vi "Teleop.vi"(10 "Match Info":T1={"Autonomous Elapsed Seconds"=0.0, "TeleOp Elapsed Seconds"=0.0, "Disabled Elapsed Seconds"=0.0, "Visited Autonomous"=FALSE, "Visited TeleOp"=FALSE, "Visited Disabled"=FALSE, "Autonomous Settings"={"Autonomous Style"=enum."Independent", "VI Refnum"=refnum}}, 11 "Call Context":T2) -> ()   [LabVIEW 2017]
doc: "This VI is called for each enabled TeleOp packet received from the DS. It is typically used to read from joysticks and other inputs and update I/O or setpoints for timed control loops. It should complete and return within 20 milliseconds or risk missing DS packets."
uses:
  <vilib>/Rock Robotics/WPI/DriverStation/WPI_DriverStationDerivedRobotMode.ctl
  <vilib>/Rock Robotics/WPI/DriverStation/WPI_DriverStationMatch Info.ctl
  <vilib>/Rock Robotics/WPI/Utilities/WPI_GetSetVariantRefNum.vi
  <vilib>/Rock Robotics/Network Tables/NT Write Boolean Array.vi
  <vilib>/Rock Robotics/Network Tables/NT Write Numeric Array.vi
  Framework/Robot Global Data.vi
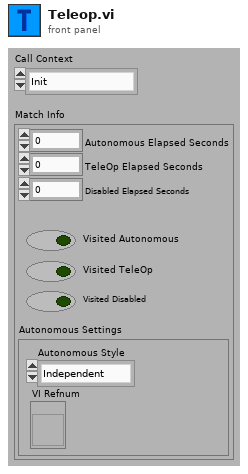
[diagram p1: front panel]
types:
  T1 = typedef "WPI_DriverStationMatch Info.ctl" = cluster{"Autonomous Elapsed Seconds":dbl, "TeleOp Elapsed Seconds":dbl, "Disabled Elapsed Seconds":dbl, "Visited Autonomous":bool, "Visited TeleOp":bool, "Visited Disabled":bool, "Autonomous Settings":cluster{"Autonomous Style":enum16{"Iterative", "Independent"}, "VI Refnum":refnum<vi>}}
  T2 = typedef "WPI_DriverStationDerivedRobotMode.ctl" = enum16{"Init", "Execute", "Stop"}
  T3 = cluster{"Grab Setpoint ":dbl, "Grab Time ":dbl, "Release Setpoint ":dbl, "Release Time ":dbl, " Button Lift Arm Setpoint ":dbl, "Button Lift Arm Time ":dbl, "Button Lower Arm Setpoint ":dbl, "Button Lower Arm Time ":dbl, "Climb Setpoint ":dbl, "Climb Time ":dbl, "Speed Rate ":dbl, "Speed Deadband ":dbl, "Turning Rate ":dbl, "Turning Deadband ":dbl}
  T4 = typedef "WPI_JoystickDevRef.ctl" = cluster{"Device":T5}
  T5 = typedef "WPI_JoystickDeviceEnum.ctl" = enum16{"USB 0", "USB 1", "USB 2", "USB 3", "USB 4", "USB 5"}
  T6 = typedef "Command Status Info.ctl" = cluster{"Name":string, "Status":T7, "notifier out":T8}
  T7 = typedef "Completion Status.ctl" = enum16{"Successful", "Aborted", "Incomplete"}
  T8 = typedef "Completion Notifier.ctl" = refnum<notifier>
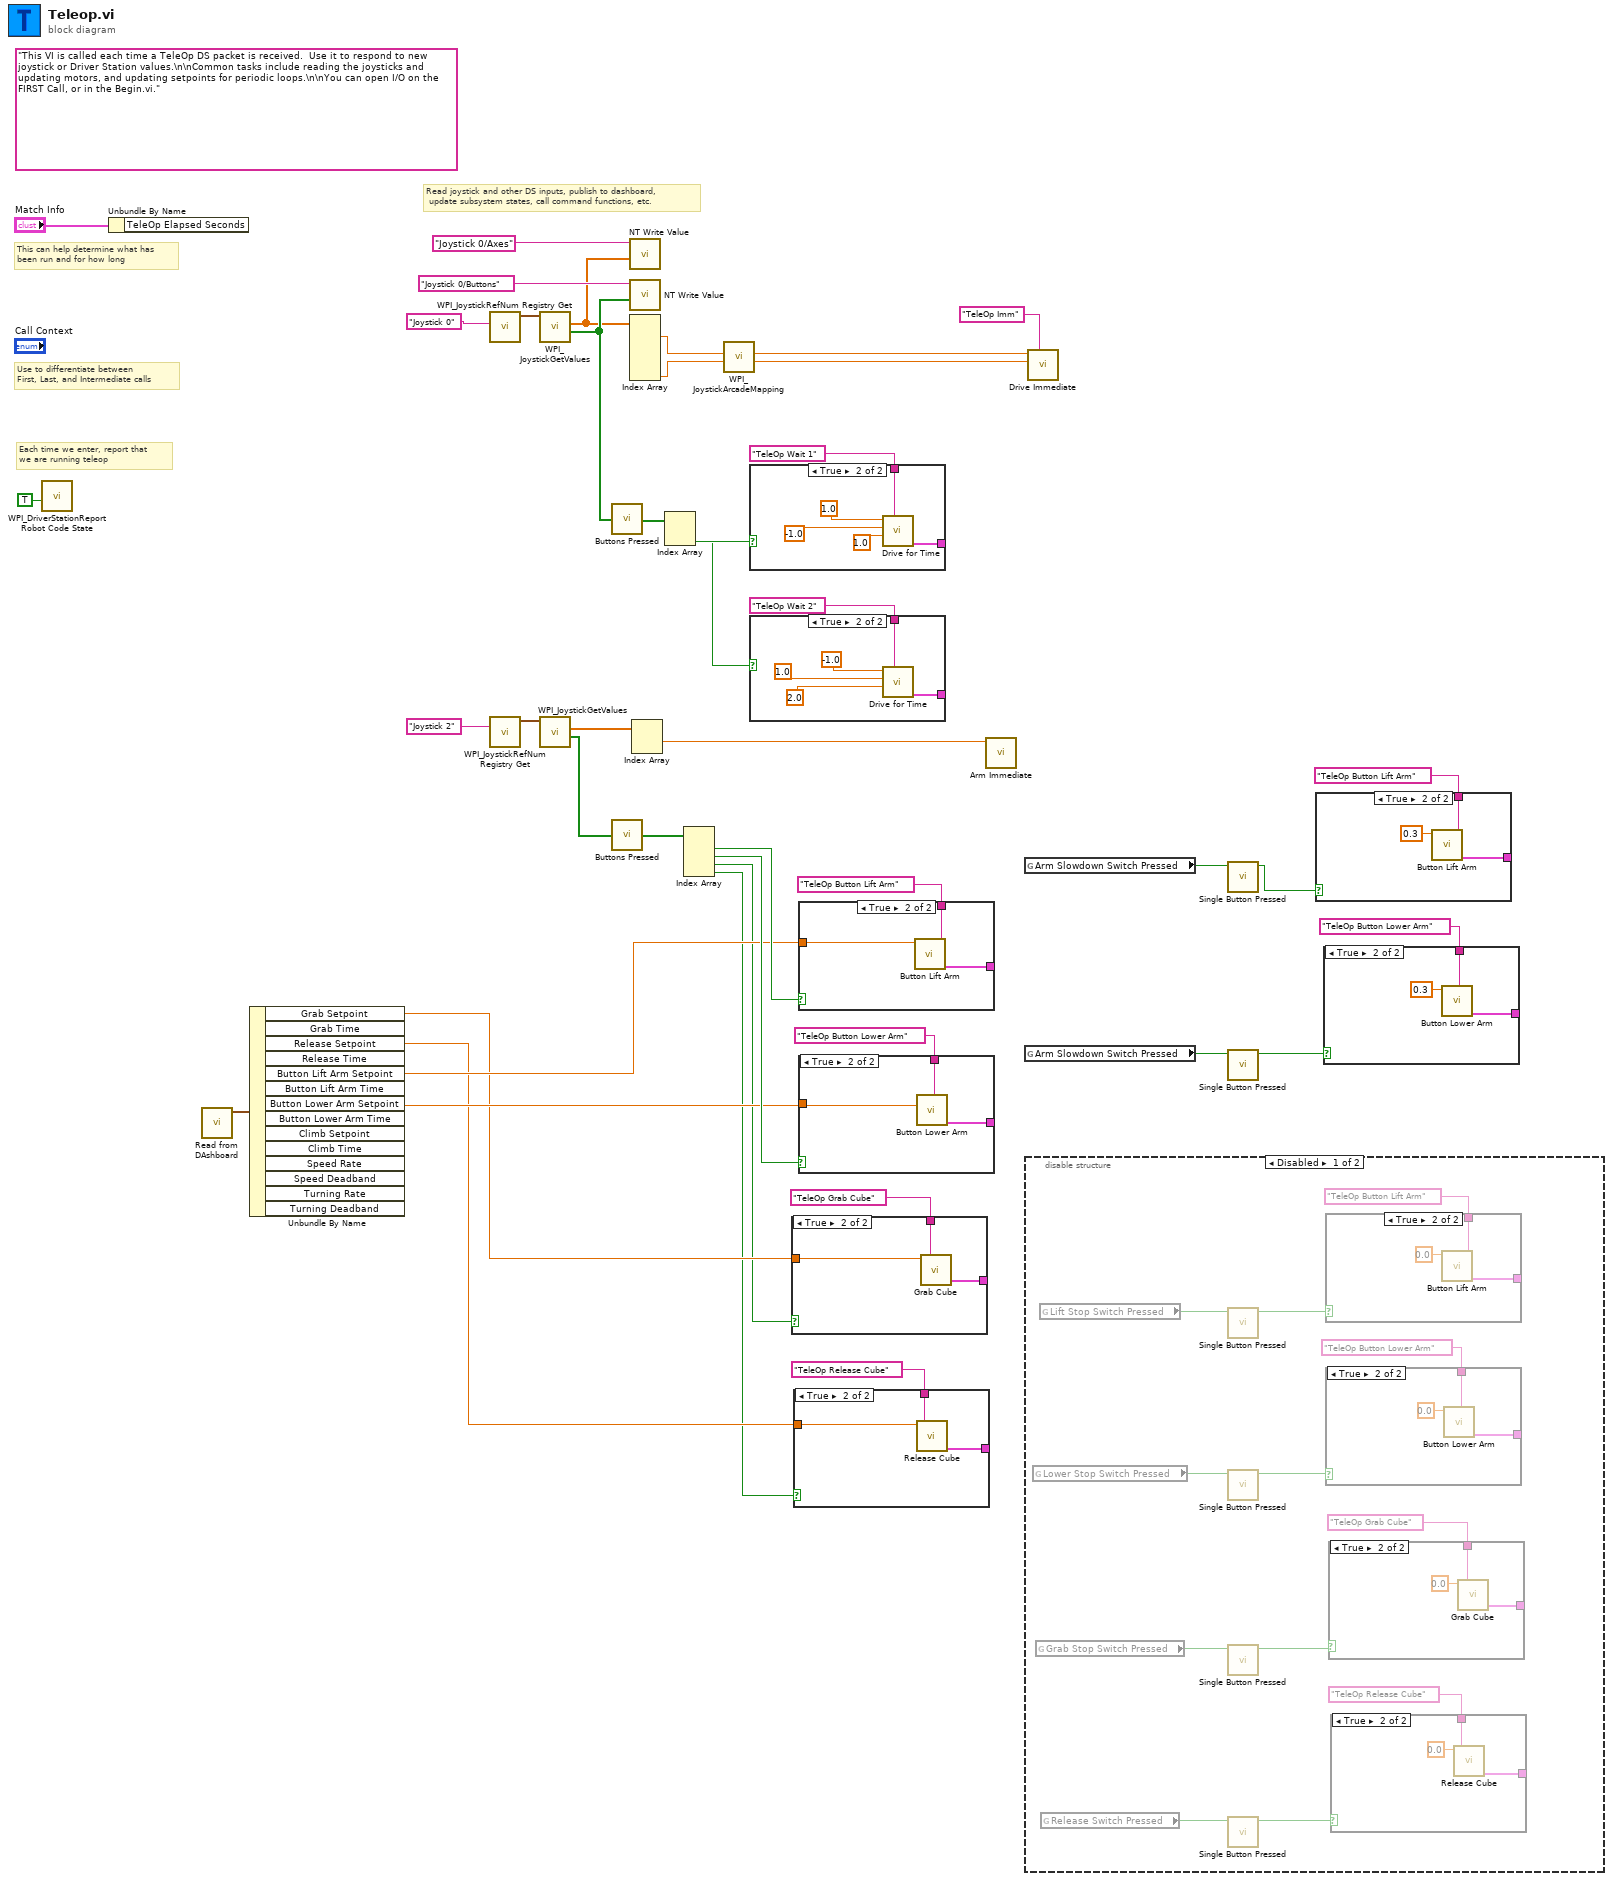
[diagram p0: block diagram]
diagram:
  (unwired) "This VI is called each time a TeleOp DS packet is received.  Use it to respond to new joystick or Driver Station values.\n\nCommon tasks include reading the joysticks and updating motors, and updating setpoints for periodic loops.\n\nYou can open I/O on the FIRST Call, or in the Begin.vi."
  # "Read joystick and other DS inputs, publish to dashboard,\n update subsystem states, call command functions, etc."
  # "Each time we enter, report that\nwe are running teleop"
  # "Use to differentiate between\nFirst, Last, and Intermediate calls"
  # "This can help determine what has\nbeen run and for how long"
  n1 = call <vilib>:"WPI_DriverStationReport Robot Code State.vi"("TeleOp"=TRUE ("Autonomous")) -> ()  [unwired: 10 in, 1 out]
  n2 = Unbundle By Name("Match Info") -> ()  [unwired: 1 out]
  n3 = call "Read from DAshboard.vi"() -> ("output cluster"=w15:T3)  [unwired: 11 in]
  n4 = Unbundle By Name(w15) -> ("Grab Setpoint"=w12:dbl, "Release Setpoint"=w11:dbl, "Button Lift Arm Setpoint"=w14:dbl, "Button Lower Arm Setpoint"=w13:dbl)  [unwired: 10 out]
  n5 = call <vilib>:"WPI_JoystickRefNum Registry Get.vi"("refnum name"="Joystick 0") -> ("JoystickDevRef"=w40:T4)  [unwired: 1 in, 9 out]
  n6 = call <vilib>:"WPI_JoystickRefNum Registry Get.vi"("refnum name"="Joystick 2") -> ("JoystickDevRef"=w25:T4)  [unwired: 1 in, 9 out]
  n7 = call <vilib>:"WPI_JoystickGetValues.vi"("JoystickDevRef"=w40) -> ("Buttons"=w31:bool[], "Axes"=w30:dbl[])  [unwired: 6 in, 3 out]
  n8 = call <vilib>:"WPI_JoystickGetValues.vi"("JoystickDevRef"=w25) -> ("Buttons"=w22:bool[], "Axes"=w24:dbl[])  [unwired: 6 in, 3 out]
  n9 = call "Buttons Pressed.vi"("Button Values"=w31) -> ("Button Presses"=w36:bool[])
  n10 = call "Buttons Pressed.vi"("Button Values"=w22) -> ("Button Presses"=w23:bool[])
  n11 = call-poly <vilib>:"NT Write Value.vi"("Numeric Array"=w30, "Name"="Joystick 0/Axes") -> ()  [unwired: 9 in, 1 out]
  n12 = call-poly <vilib>:"NT Write Value.vi"("Boolean Array"=w31, "Name"="Joystick 0/Buttons") -> ()  [unwired: 9 in, 1 out]
  n13 = Index Array(array=w30) -> (element #1=w33:dbl, element #6=w2:dbl)  [unwired: 6 in, 4 out]
  n14 = Index Array(array=w24) -> (element #1=w1:dbl)  [unwired: 2 in, 1 out]
  n15 = Index Array(array=w36) -> (element #1=w35:bool, element #2=w34:bool)  [unwired: 2 in]
  n16 = Index Array(array=w23) -> (element #1=w21:bool, element #2=w19:bool, element #3=w10:bool, element #4=w9:bool)  [unwired: 4 in]
  n17 = call <vilib>:"WPI_JoystickArcadeMapping.vi"("Y axis value"=w2, "X axis value"=w33) -> ("Right Motor Value"=w27:dbl, "Left Motor Value"=w28:dbl)  [unwired: 8 in]
  n18 = case shown="True" w35 {
    tunnel: [_ w47] -> _
    tunnel: "TeleOp Wait 1" ("Description") -> [_ w46]
    frame False {
    }
    frame True {
      n19 = call "Drive for Time.vi"("Description"=w46, "Seconds"=1.0, "Right Speed"=-1.0, "Left Speed"=1.0) -> ("Command Info Out"=w47:T6)  [unwired: 6 in, 1 out]
    }
  }
  n20 = case shown="True" w34 {
    tunnel: [_ w51] -> _
    tunnel: "TeleOp Wait 2" ("Description") -> [_ w50]
    frame False {
    }
    frame True {
      n21 = call "Drive for Time.vi"("Description"=w50, "Seconds"=2.0, "Right Speed"=1.0, "Left Speed"=-1.0) -> ("Command Info Out"=w51:T6)  [unwired: 6 in, 1 out]
    }
  }
  n22 = case shown="True" w10 {
    tunnel: "TeleOp Grab Cube" ("Description") -> [_ w56]
    tunnel: [_ w55] -> _
    tunnel: w12 -> [_ w54]
    frame False {
    }
    frame True {
      n23 = call "Grab Cube.vi"("Description"=w56, "Setpoint"=w54) -> ("Command Info Out"=w55:T6)  [unwired: 9 in]
    }
  }
  n24 = case shown="True" w9 {
    tunnel: "TeleOp Release Cube" ("Description") -> [_ w59]
    tunnel: [_ w58] -> _
    tunnel: w11 -> [_ w57]
    frame False {
    }
    frame True {
      n25 = call "Release Cube.vi"("Description"=w59, "Setpoint"=w57) -> ("Command Info Out"=w58:T6)  [unwired: 9 in]
    }
  }
  n26 = case shown="True" w21 {
    tunnel: "TeleOp Button Lift Arm" ("Description") -> [_ w62]
    tunnel: [_ w61] -> _
    tunnel: w14 -> [_ w60]
    frame False {
    }
    frame True {
      n27 = call "Button Lift Arm.vi"("Description"=w62, "Setpoint"=w60) -> ("Command Info Out"=w61:T6)  [unwired: 9 in]
    }
  }
  n28 = case shown="True" w19 {
    tunnel: "TeleOp Button Lower Arm" ("Description") -> [_ w65]
    tunnel: [_ w64] -> _
    tunnel: w13 -> [_ w63]
    frame False {
    }
    frame True {
      n29 = call "Button Lower Arm.vi"("Description"=w65, "Setpoint"=w63) -> ("Command Info Out"=w64:T6)  [unwired: 9 in]
    }
  }
  n30 = call "Arm Immediate.vi"("Setpoint"=w1) -> ()  [unwired: 10 in, 1 out]
  n31 = global read "Robot Global Data.vi" "Arm Slowdown Switch Pressed"() -> (w8:bool)
  n32 = global read "Robot Global Data.vi" "Arm Slowdown Switch Pressed"() -> (w4:bool)
  n33 = disable-structure shown="Disabled" {
    frame Disabled {
      n34 = global read "Robot Global Data.vi" "Lower Stop Switch Pressed"() -> (w72:bool)
      n35 = global read "Robot Global Data.vi" "Grab Stop Switch Pressed"() -> (w71:bool)
      n36 = global read "Robot Global Data.vi" "Lift Stop Switch Pressed"() -> (w73:bool)
      n37 = global read "Robot Global Data.vi" "Release Switch Pressed"() -> (w70:bool)
      n38 = call "Single Button Pressed.vi"("Button Value"=w73) -> ("Button Press"=w66:bool)  [unwired: 10 in]
      n39 = call "Single Button Pressed.vi"("Button Value"=w72) -> ("Button Press"=w67:bool)  [unwired: 10 in]
      n40 = call "Single Button Pressed.vi"("Button Value"=w71) -> ("Button Press"=w68:bool)  [unwired: 10 in]
      n41 = call "Single Button Pressed.vi"("Button Value"=w70) -> ("Button Press"=w69:bool)  [unwired: 10 in]
      n42 = case shown="True" w66 {
        tunnel: "TeleOp Button Lift Arm" ("Description") -> [_ w89]
        tunnel: [_ w88] -> _
        frame False {
        }
        frame True {
          n43 = call "Button Lift Arm.vi"("Description"=w89, "Setpoint"=0.0) -> ("Command Info Out"=w88:T6)  [unwired: 9 in]
        }
      }
      n44 = case shown="True" w67 {
        tunnel: "TeleOp Button Lower Arm" ("Description") -> [_ w86]
        tunnel: [_ w85] -> _
        frame False {
        }
        frame True {
          n45 = call "Button Lower Arm.vi"("Description"=w86, "Setpoint"=0.0) -> ("Command Info Out"=w85:T6)  [unwired: 9 in]
        }
      }
      n46 = case shown="True" w68 {
        tunnel: "TeleOp Grab Cube" ("Description") -> [_ w83]
        tunnel: [_ w82] -> _
        frame False {
        }
        frame True {
          n47 = call "Grab Cube.vi"("Description"=w83, "Setpoint"=0.0) -> ("Command Info Out"=w82:T6)  [unwired: 9 in]
        }
      }
      n48 = case shown="True" w69 {
        tunnel: "TeleOp Release Cube" ("Description") -> [_ w80]
        tunnel: [_ w79] -> _
        frame False {
        }
        frame True {
          n49 = call "Release Cube.vi"("Description"=w80, "Setpoint"=0.0) -> ("Command Info Out"=w79:T6)  [unwired: 9 in]
        }
      }
    }
    frame Enabled {
    }
  }
  n50 = call "Drive Immediate.vi"("Description"="TeleOp Imm", "Right Setpoint"=w27, "Left Setpoint"=w28) -> ()  [unwired: 8 in, 1 out]
  n51 = call "Single Button Pressed.vi"("Button Value"=w8) -> ("Button Press"=w6:bool)  [unwired: 10 in]
  n52 = call "Single Button Pressed.vi"("Button Value"=w4) -> ("Button Press"=w3:bool)  [unwired: 10 in]
  n53 = case shown="True" w6 {
    tunnel: "TeleOp Button Lift Arm" ("Description") -> [_ w92]
    tunnel: [_ w91] -> _
    frame False {
    }
    frame True {
      n54 = call "Button Lift Arm.vi"("Description"=w92, "Setpoint"=0.3) -> ("Command Info Out"=w91:T6)  [unwired: 9 in]
    }
  }
  n55 = case shown="True" w3 {
    tunnel: "TeleOp Button Lower Arm" ("Description") -> [_ w95]
    tunnel: [_ w94] -> _
    frame False {
    }
    frame True {
      n56 = call "Button Lower Arm.vi"("Description"=w95, "Setpoint"=0.3) -> ("Command Info Out"=w94:T6)  [unwired: 9 in]
    }
  }
